vi "GenerateAbsorptionCrossSectionsFromRIandCalibrationCurve.vi"(9 "Offset":dbl, 10 "slope":dbl, 11 "Extinction ExtinctionUncertainity Size parameter and Number of sizes input":T1={"PAS amplitude"=[1.9915476e-09, 2.5260327e-09, 2.9463496e-09, 3.6659398e-09, 4.1150909e-09, 4.3561701e-09, 4.8158371e-09, 5.5805258e-09], "PAS amp Uncertainty"=[1.1685435e-10, 1.8562181e-10, 2.4682015e-10, 3.9807269e-10, 5.4913102e-10, 1.091901e-09, 1.2235488e-09, 1.7175431e-09], "Size parameters"=[2.4744035643168516, 2.699349342891111, 2.92429512146537, 3.149240900039629, 3.3741866786138885, 3.599132457188148, 3.8240782357624066, 4.049024014336666], "Number ofSizes"=8.0, "GeometricCrossSection"=[5.939573610693203e-10, 7.068583470577035e-10, 8.295768100885549e-10, 9.621127501618742e-10, 1.1044661672776617e-09, 1.2566370614359174e-09, 1.418625432636641e-09, 1.590431280879833e-09], "Wave Length"=349.14999, "SMPS Sizes"=[105.5, 109.4, 113.4, 117.6, 121.9, 126.3, 131.0, 135.8, 140.7, 145.9, 151.2, 156.8, 162.5, 168.5, 174.7, 181.1, 187.7, 194.6, 201.7, 209.1, 216.7, 224.7, 232.9, 241.4, 250.3, 259.5, 269.0, 278.8, 289.0, 299.6, 310.6, 322.0, 333.8, 346.0, 358.7, 371.8, 385.4, 399.5, 414.2, 429.4, 445.1, 461.4, 478.3, 495.8, 514.0, 532.8, 552.3, 572.5, 593.5, 615.3, 637.8, 661.2, 685.4, 710.5, 736.5, 763.5, 791.5], "Concentration"=array8x57[456 elements], "Double Charge Correction"=TRUE, "Extincation Factor"=1.0, "Diameter Factor"=1.0, "Diameter Offset"=0.0, "Extinction Factor Flag"=FALSE, "Diameter Factor Flag"=FALSE, "Diameter Offset Flag"=FALSE, "Sizes"=[275.0, 300.0, 325.0, 350.0, 375.0, 400.0, 425.0, 450.0], "ExtinctionOrAbsorptionOrScattering"=0, "Concentration(#/cc)"=[]} {"ExtinctionOrAbsorptionOrScattering" scale=0.0..2.0}) -> (3 "Extinction ExtinctionUncertainity Size parameter and Number ofS sizes outpu":T1={"PAS amplitude"=[1.9915476e-09, 2.5260327e-09, 2.9463496e-09, 3.6659398e-09, 4.1150909e-09, 4.3561701e-09, 4.8158371e-09, 5.5805258e-09], "PAS amp Uncertainty"=[1.1685435e-10, 1.8562181e-10, 2.4682015e-10, 3.9807269e-10, 5.4913102e-10, 1.091901e-09, 1.2235488e-09, 1.7175431e-09], "Size parameters"=[2.4744035643168516, 2.699349342891111, 2.92429512146537, 3.149240900039629, 3.3741866786138885, 3.599132457188148, 3.8240782357624066, 4.049024014336666], "Number ofSizes"=8.0, "GeometricCrossSection"=[5.939573610693203e-10, 7.068583470577035e-10, 8.295768100885549e-10, 9.621127501618742e-10, 1.1044661672776617e-09, 1.2566370614359174e-09, 1.418625432636641e-09, 1.590431280879833e-09], "Wave Length"=349.14999, "SMPS Sizes"=[105.5, 109.4, 113.4, 117.6, 121.9, 126.3, 131.0, 135.8, 140.7, 145.9, 151.2, 156.8, 162.5, 168.5, 174.7, 181.1, 187.7, 194.6, 201.7, 209.1, 216.7, 224.7, 232.9, 241.4, 250.3, 259.5, 269.0, 278.8, 289.0, 299.6, 310.6, 322.0, 333.8, 346.0, 358.7, 371.8, 385.4, 399.5, 414.2, 429.4, 445.1, 461.4, 478.3, 495.8, 514.0, 532.8, 552.3, 572.5, 593.5, 615.3, 637.8, 661.2, 685.4, 710.5, 736.5, 763.5, 791.5], "Concentration"=array8x57[456 elements], "Double Charge Correction"=TRUE, "Extincation Factor"=1.0, "Diameter Factor"=1.0, "Diameter Offset"=0.0, "Extinction Factor Flag"=FALSE, "Diameter Factor Flag"=FALSE, "Diameter Offset Flag"=FALSE, "Sizes"=[275.0, 300.0, 325.0, 350.0, 375.0, 400.0, 425.0, 450.0], "ExtinctionOrAbsorptionOrScattering"=0, "Concentration(#/cc)"=[]} {"ExtinctionOrAbsorptionOrScattering" scale=0.0..2.0})   [LabVIEW 2013]
uses:
  BaesDataTypeDefinition.ctl
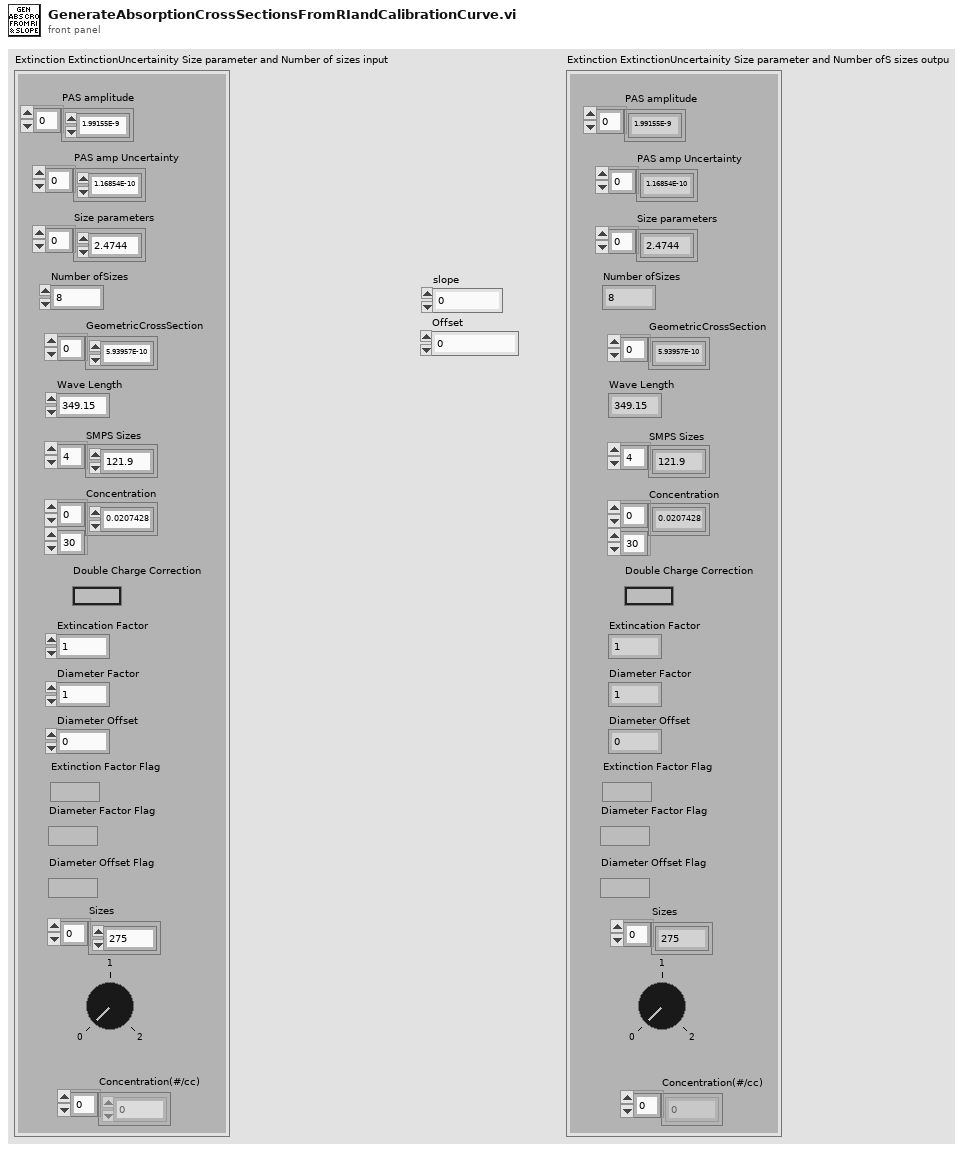
[diagram p1: front panel]
types:
  T1 = typedef "BaesDataTypeDefinition.ctl" = cluster{"PAS amplitude":dbl[], "PAS amp Uncertainty":dbl[], "Size parameters":dbl[], "Number ofSizes":dbl, "GeometricCrossSection":dbl[], "Wave Length":dbl, "SMPS Sizes":dbl[], "Concentration":dbl[][], "Double Charge Correction":bool, "Extincation Factor":dbl, "Diameter Factor":dbl, "Diameter Offset":dbl, "Extinction Factor Flag":bool, "Diameter Factor Flag":bool, "Diameter Offset Flag":bool, "Sizes":dbl[], "ExtinctionOrAbsorptionOrScattering":i8, "Concentration(#/cc)":dbl[]}
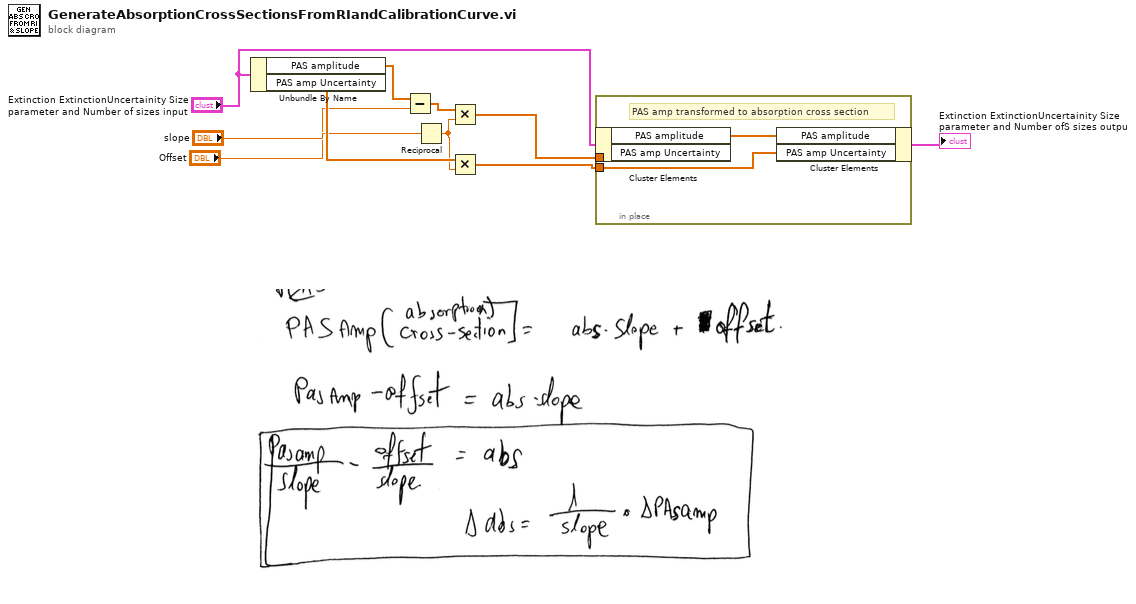
[diagram p0: block diagram]
diagram:
  n1 = Unbundle By Name("Extinction ExtinctionUncertainity Size parameter and Number of sizes input") -> ("PAS amplitude"=w10:dbl[], "PAS amp Uncertainty"=w8:dbl[])
  n2 = Subtract(x=w10, y="Offset") -> (x-y=w9:dbl[])
  n3 = Reciprocal(x="slope") -> (1/x=w7:dbl)
  n4 = Multiply(x=w9, y=w7) -> (x*y=w4:dbl[])
  n5 = Multiply(x=w8, y=w7) -> (x*y=w3:dbl[])
  n6 = in-place {
    in-place-border: w4 -> [w12]
    in-place-border: w3 -> [w11]
    # "PAS amp transformed to absorption cross section"
    n7 = in-place-cluster #1("Extinction ExtinctionUncertainity Size parameter and Number of sizes input") -> ()  [unwired: 2 out]
    n8 = in-place-cluster #1("PAS amplitude"=w12, "PAS amp Uncertainty"=w11) -> (→"Extinction ExtinctionUncertainity Size parameter and Number ofS sizes outpu":T1)
  }
